vi "Keithley Sweep and Acquire Measurements.vi"(4 "Source Delay (s)":dbl=0.1, 5 "Sweep Direction":u16(ring) items=["Low to high", "High to low"], 6 "Number of Points":u32=5, 7 "Maximum Amplitude":dbl=2.0, 8 "Minimum Amplitude":dbl=1.0, 9 "VISA resource name":refnum<visa-resource-name>) -> (0 "Measurement Complete":bool, 2 "Data Array":dbl[][](array[numeric]), 3 "VISA resource name out":refnum<visa-resource-name>)   [LabVIEW 2011]
doc: "Configures a sweep and takes voltage and current readings at each point."
uses:
  <instrlib>/Keithley 24XX/Public/Data/Read (Multiple Points).vi
  <instrlib>/Keithley 24XX/Keithley 24XX.lvlib
panel:
  out "XY Graph":cluster{"Voltage":sgl[], "Current":sgl[]}(graph)
  in  "Source Mode  (0: Voltage)":u16(ring) items=["Voltage", "Current"]
  in  "Timeout (10000 ms)":i32=60000 format="%#.6g"
  in  "Compliance  Level":dbl=0.1
  # "(c) 2006 National Instruments.  ALL RIGHTS RESERVED."
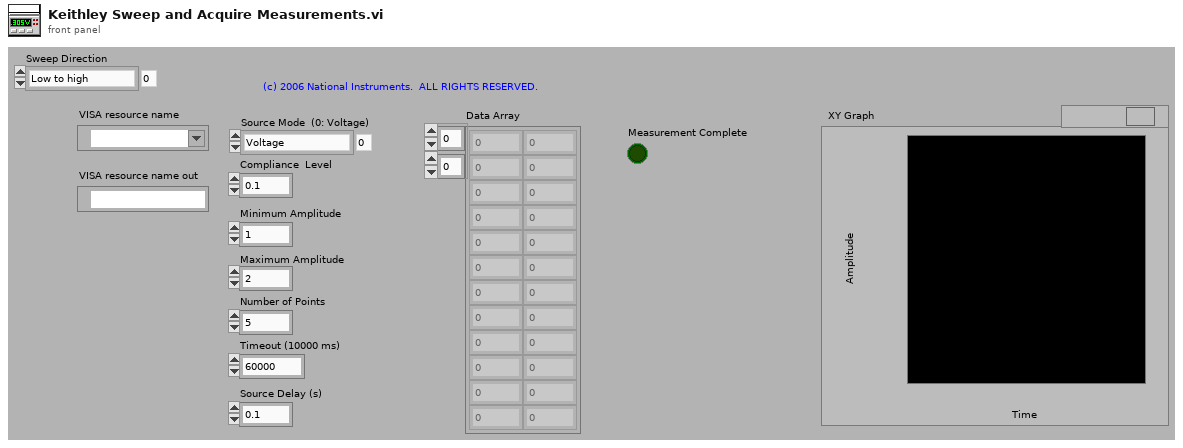
[diagram p1: front panel]
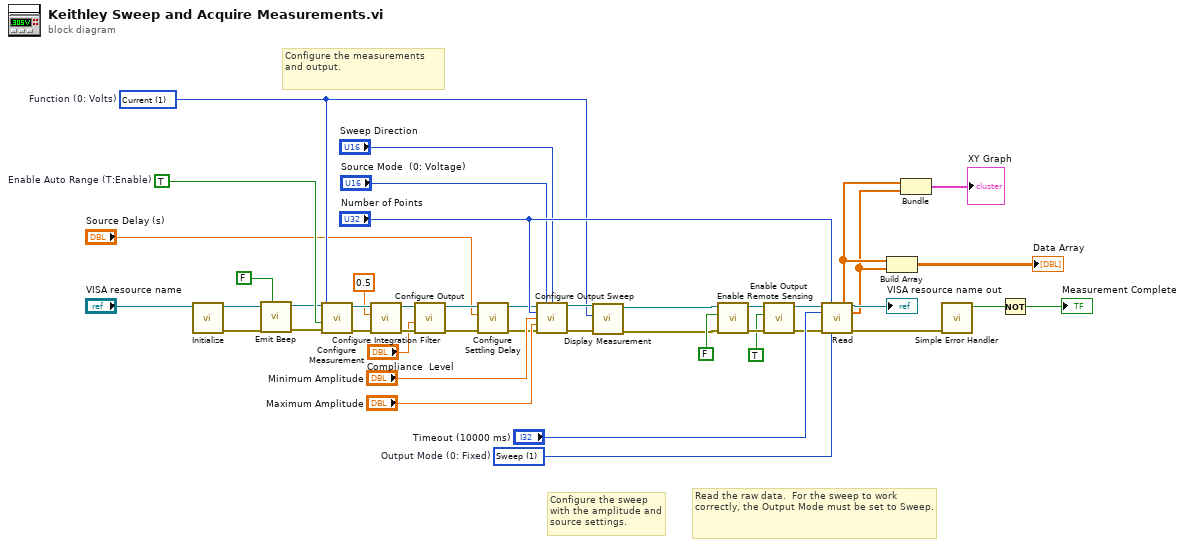
[diagram p0: block diagram]
diagram:
  w36 = TRUE  # Enable Auto Range (T:Enable)
  w20 = u16 1 items=["Volts", "Current", "Resistance"]  # Function (0: Volts)
  w39 = u16 1 items=["Fixed", "Sweep", "List"]  # Output Mode (0: Fixed)
  # "Read the raw data.  For the sweep to work correctly, the Output Mode must be set to Sweep."
  # "Configure the sweep with the amplitude and source settings."
  # "Configure the measurements and output."
  n1 = call <instrlib>:"Initialize.vi"("VISA resource name"="VISA resource name") -> ("error out"=w8:errorcluster, "VISA resource name out"=w11:refnum<visa-resource-name>)  [unwired: 9 in]
  n2 = call <instrlib>:"Emit Beep.vi"("Enable Beep (F)"=FALSE, "error in (no error)"=w8, "VISA resource name"=w11) -> ("error out"=w9:errorcluster, "VISA resource name out"=w10:refnum<visa-resource-name>)  [unwired: 7 in]
  n3 = call <instrlib>:"Configure Measurement.vi"("error in (no error)"=w9, "Enable Auto Range (T:Enable)"=w36, "Function (0: Volts)"=w20, "VISA resource name"=w10) -> ("error out"=w23:errorcluster, "VISA resource name out"=w24:refnum<visa-resource-name>)  [unwired: 6 in]
  n4 = call <instrlib>:"Configure Integration Filter.vi"("error in (no error)"=w23, "Measurement Speed (1 PLC)"=0.5, "VISA resource name"=w24) -> ("error out"=w18:errorcluster, "VISA resource name out"=w19:refnum<visa-resource-name>)  [unwired: 7 in]
  n5 = call <instrlib>:"Configure Output.vi"("error in (no error)"=w18, "Compliance  Level (0.1)"="Compliance  Level", "VISA resource name"=w19) -> ("error out"=w15:errorcluster, "VISA resource name out"=w16:refnum<visa-resource-name>)  [unwired: 7 in]
  n6 = call <instrlib>:"Configure Settling Delay.vi"("error in (no error)"=w15, "Manual Settling Delay (0 sec)"="Source Delay (s)", "VISA resource name"=w16) -> ("error out"=w13:errorcluster, "VISA resource name out"=w14:refnum<visa-resource-name>)  [unwired: 7 in]
  n7 = call <instrlib>:"Configure Output Sweep.vi"("VISA resource name"=w14, "Source Mode  (0: Voltage)"="Source Mode  (0: Voltage)", "Sweep Direction  (0: Ascending)"="Sweep Direction", "Number of Points (5)"="Number of Points", "Minimum Amplitude (1)"="Minimum Amplitude", "Maximum Amplitude (2)"="Maximum Amplitude", "error in (no error)"=w13) -> ("VISA resource name out"=w22:refnum<visa-resource-name>, "error out"=w21:errorcluster)  [unwired: 7 in]
  n8 = call <instrlib>:"Display Measurement.vi"("error in (no error)"=w21, "Displayed Measurement (0: Voltage)"=w20, "VISA resource name"=w22) -> ("error out"=w5:errorcluster, "VISA resource name out"=w6:refnum<visa-resource-name>)  [unwired: 7 in]
  n9 = call <instrlib>:"Enable Remote Sensing.vi"("error in (no error)"=w5, "Enable Remote Sensing (T: Enable)"=FALSE ("Enable Output (T: Enable)"), "VISA resource name"=w6) -> ("error out"=w28:errorcluster, "VISA resource name out"=w29:refnum<visa-resource-name>)  [unwired: 7 in]
  n10 = call <instrlib>:"Enable Output.vi"("error in (no error)"=w28, "Enable Output (T: Enable)"=TRUE, "VISA resource name"=w29) -> ("error out"=w38:errorcluster, "VISA resource name out"=w37:refnum<visa-resource-name>)  [unwired: 7 in]
  n11 = call-poly <instrlib>:"Read.vi"("VISA resource name"=w37, "Sample Count (1)"="Number of Points", "Timeout (10000 ms)"="Timeout (10000 ms)", "error in (no error)"=w38, "Output Mode (0: Fixed)"=w39) -> ("Voltage"=w3:sgl[], "VISA resource name out"=→"VISA resource name out":refnum<visa-resource-name>, "Current"=w2:sgl[], "error out"=w34:errorcluster)  [unwired: 4 in, 3 out]
  n12 = Build Array(w3, w2) -> (→"Data Array":sgl[][])
  n13 = Bundle("Voltage"=w3, "Current"=w2) -> (→"XY Graph":cluster{"Voltage":sgl[], "Current":sgl[]})  [unwired: 1 in]
  n14 = call <vilib>:"Simple Error Handler.vi"("error in (no error)"=w34) -> ("error?"=w32:bool)  [unwired: 4 in, 4 out]
  n15 = Not(x=w32) -> (.not. x?=→"Measurement Complete":bool)
